vi "FTW-Message-Actor-Interpret.vi"(8 "error in":errorcluster, 11 "Message":refnum<class "FTW-Message.lvclass">) -> (0 "error out":errorcluster, 1 "Sender":string, 2 "Parameter":string, 3 "Payload":variant)   [LabVIEW 2014, in "FTW-Message-Actor.lvclass"]
uses:
  FTW-Message-Actor.lvclass
  Message/FTW-Message.lvclass
panel:
  # "Inputs"
  # "Outputs"
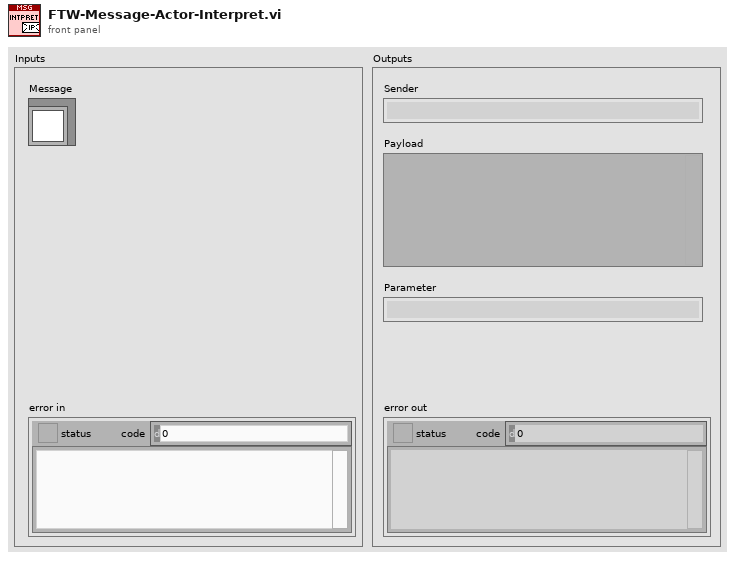
[diagram p1: front panel]
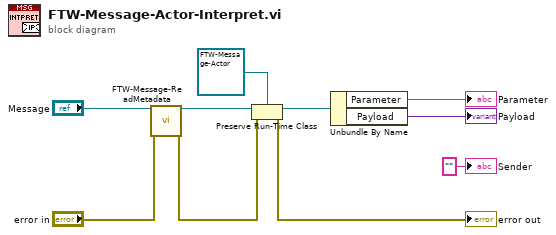
[diagram p0: block diagram]
diagram:
  n1 = call "FTW-Message-ReadMetadata.vi"("Message"="Message", "error in"="error in") -> ("Message out"=w8:refnum<class "FTW-Message.lvclass">, "error out"=w6:errorcluster)  [unwired: 10 in, 2 out]
  n2 = Preserve Run-Time Class(object in=w8, error in=w6, 2:refnum<class "FTW-Message-Actor.lvclass"> refnum ("Actor Message")) -> (object out=w4:refnum<class "FTW-Message-Actor.lvclass">, error out=→"error out":errorcluster)
  n3 = Unbundle By Name(w4) -> ("Parameter"=→"Parameter":string, "Payload"=→"Payload":variant)
  "Sender" <- "" ("Sender")
